vi "Get ALL.vi"(11 "Created Info in":refnum<class "Created Info.lvclass">) -> (0 "Implemented Msgs":T1, 1 "Is Normal":bool, 2 "Self":refnum<user-event>)   [LabVIEW 2021, in "jettl.lvlib" / "Actor.lvlib" / "Created Info.lvclass"]
uses:
  Created Info.lvclass
  Msg/Msg.lvclass
  Utilities/Implemented Msgs.ctl
  Created Info.lvclass/Created Info.ctl
  Utilities/Utilities.lvlib
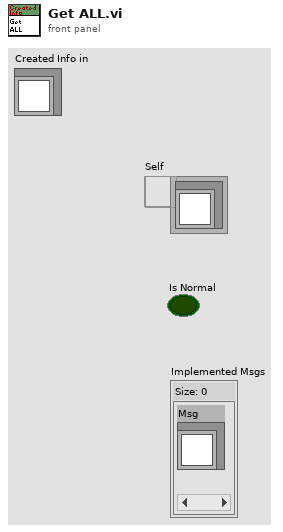
[diagram p1: front panel]
types:
  T1 = typedef "jettl.lvlib/Utilities.lvlib/Implemented Msgs.ctl" = set{refnum<class "Msg.lvclass">}
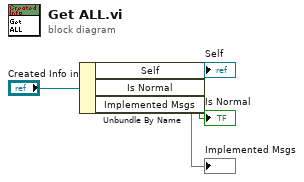
[diagram p0: block diagram]
diagram:
  n1 = Unbundle By Name("Created Info in") -> ("Self"=→"Self":refnum<user-event>, "Is Normal"=→"Is Normal":bool, "Implemented Msgs"=→"Implemented Msgs":T1)
